vi "Update Animation.vi"(11 "Chmmr in":refnum<class "Chmmr.lvclass">) -> (3 "Chmmr out":refnum<class "Chmmr.lvclass">)   [LabVIEW 2021, in "Chmmr.lvclass"]
uses:
  Chmmr.lvclass
  Chmmr.lvclass/Chmmr.ctl
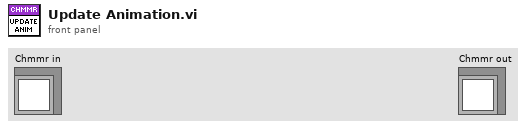
[diagram p1: front panel]
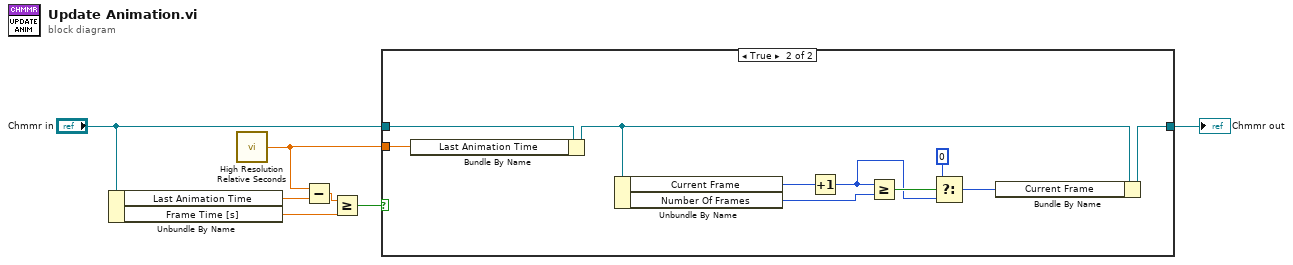
[diagram p0: block diagram]
diagram:
  n1 = Unbundle By Name("Chmmr in") -> ("Last Animation Time"=w5:dbl, "Frame Time [s]"=w7:dbl)
  n2 = call <vilib>:"High Resolution Relative Seconds.vi"() -> ("relative seconds"=w1:dbl)
  n3 = Subtract(x=w1, y=w5) -> (x-y=w6:dbl)
  n4 = Greater Or Equal?(x=w6, y=w7) -> (x >= y?=w2:bool)
  n5 = case shown="True" w2 {
    tunnel: [w8 w16] -> w3
    tunnel: "Chmmr in" -> [w8 w18]
    tunnel: w1 -> [_ w9]
    frame False {
    }
    frame True {
      n6 = Bundle By Name(cluster=w18, "Last Animation Time"=w9) -> (w17:refnum<class "Chmmr.lvclass">)
      n7 = Unbundle By Name(w17) -> ("Current Frame"=w14:i32, "Number Of Frames"=w13:i32)
      n8 = Increment(x=w14) -> (x+1=w10:i32)
      n9 = Greater Or Equal?(x=w10, y=w13) -> (x >= y?=w12:bool)
      n10 = Select(t=0, s=w12, f=w10) -> (s? t:f=w15:i32)
      n11 = Bundle By Name(cluster=w17, "Current Frame"=w15) -> (w16:refnum<class "Chmmr.lvclass">)
    }
  }
  "Chmmr out" <- w3
